vi "g_MicroZed_Interface.vi"() -> ()   [LabVIEW 2014]
uses:
  c_MicroZedInstr_Enum.ctl
panel:
  in  "Parameters":string
  in  "Run Timer":bool
  out "Test Timeout":bool
  out "Busy":bool
  out "Terminal":string
  out "read buffer":string
  in  "Start":bool
  in  "Command":T1
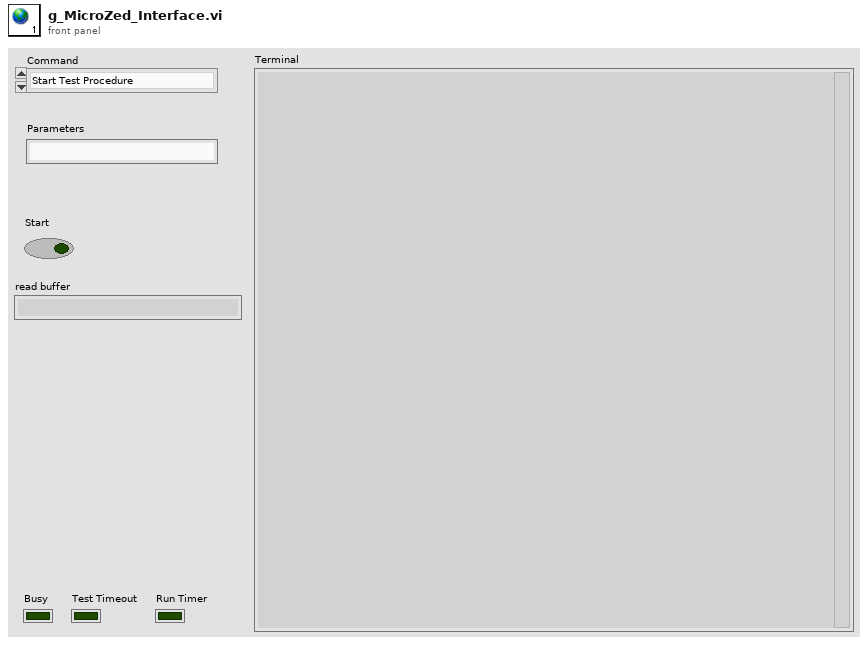
[diagram p1: front panel]
types:
  T1 = typedef "c_MicroZedInstr_Enum.ctl" = enum16{"Start Test Procedure", "Print Instructions", "Config HCC Register", "Send Parameters"}
diagram:
